vi "Tree -- Cron Library.vi"() -> ()   [LabVIEW 2013]
uses:
  JobReport/JobReport.lvclass
  JobReport/JobReport.lvclass/JobReport.ctl
  Job/Job Report -- cluster.ctl
  Job/Job.lvclass
  Job/Job.lvclass/Job.ctl
  Cron.Quartz/Cron.Quartz.lvclass
  Cron.Unix/Cron.Unix.lvclass
  Cron.Jenkins/Cron.Jenkins.lvclass
  Cron/Cron.lvclass/Cron.ctl
  Job/Read Abort Notifier.vi
  <vilib>/Utility/error.llb/Error Cluster From Error Code.vi
  Cron/Cron.lvclass
  openCron.lvlib
  Job.StaticVIRef/Job.StaticVIRef.lvclass
panel:
  out "Next Occurence 3":timestamp
  out "syntax valid? (Jenkins)":bool
  out "Next Occurence 2":timestamp
  out "syntax valid? (Unix)":bool
  out "syntax valid? (Quartz)":bool
  out "Next Occurence":timestamp
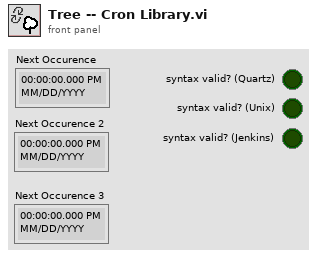
[diagram p1: front panel]
types:
  T1 = typedef "openCronJob.lvlib/JobReport.lvclass/Job Report -- cluster.ctl" = cluster{"Name":string, "GUID":string, "Start Time":timestamp, "Duration (s)":dbl, "exception code":i32, "stdin":string, "stdout":string}
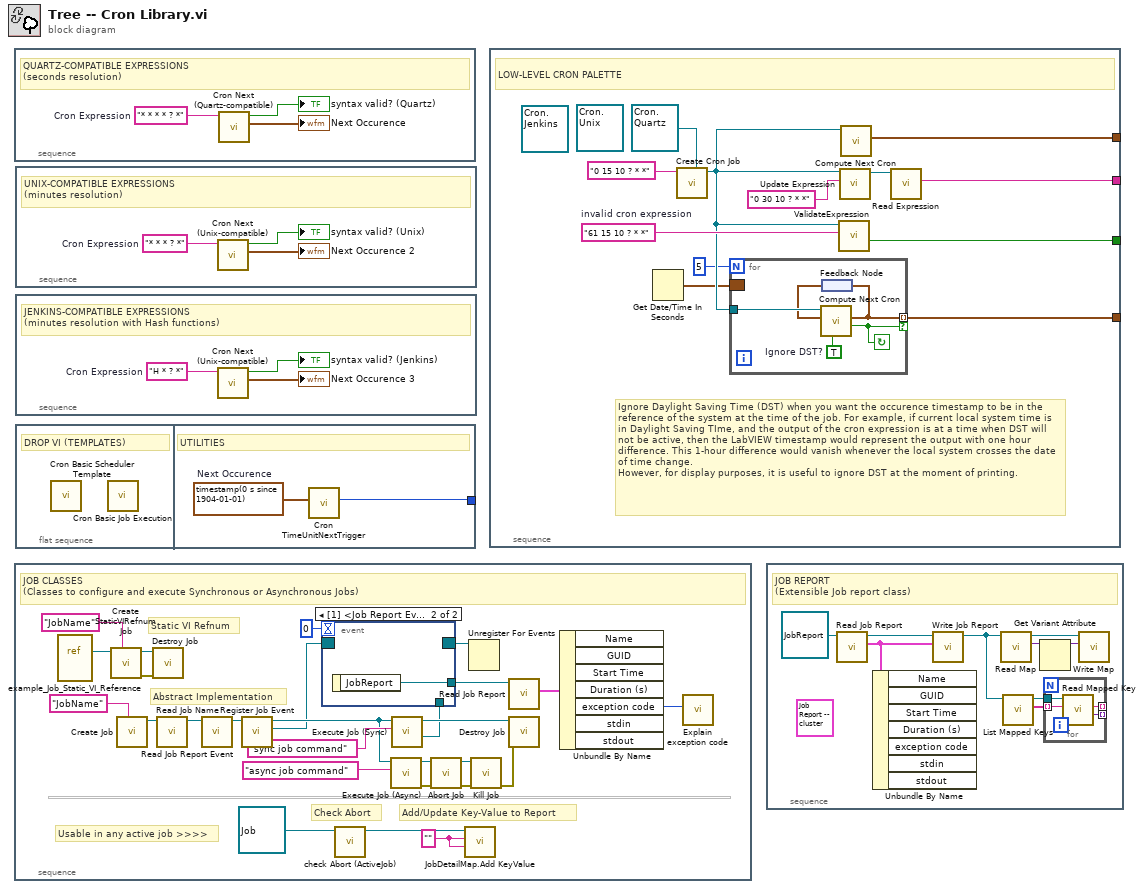
[diagram p0: block diagram]
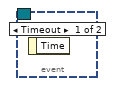
[diagram p2: hidden frame]
diagram:
  n1 = stacked-sequence {
    frame #0 {
      w3 = "* * * * ? *"  # Cron Expression
      # "QUARTZ-COMPATIBLE EXPRESSIONS\n(seconds resolution)"
      n2 = call "Cron Next (Quartz-compatible).vi"("Cron Expression"=w3) -> ("Next Occurence"=→"Next Occurence":timestamp, "syntax valid?"=→"syntax valid? (Quartz)":bool)  [unwired: 8 in, 1 out]
    }
  }
  n3 = stacked-sequence {
    frame #0 {
      w4 = "" ("Key")
      # "Add/Update Key-Value to Report"
      # "Check Abort"
      # "Usable in any active job >>>>"
      # "Abstract Implementation"
      # "Static VI Refnum"
      # "JOB CLASSES\n(Classes to configure and execute Synchronous or Asynchronous Jobs)"
      n4 = vi-ref "example_Job_Static_VI_Reference.vi"() -> (w14:refnum<vi>)
      n5 = call "Create StaticVIRefnum Job.vi"("Job Name"="JobName", "Static VI Refnum"=w14) -> ("error out"=w15:errorcluster, "Job.StaticVIRef out"=w16:refnum<class "Job.StaticVIRef.lvclass">)  [unwired: 8 in]
      n6 = call "Create Job.vi"("Job Name"="JobName") -> ("Job"=w29:refnum<class "Job.lvclass">)  [unwired: 9 in, 1 out]
      n7 = call "Destroy Job.vi"("error in (no error)"=w15, "Job in"=w16) -> ()  [unwired: 8 in, 2 out]
      n8 = call "Read Job Name.vi"("Job in"=w29) -> ("Job out"=w25:refnum<class "Job.lvclass">)  [unwired: 8 in, 2 out]
      n9 = call "Read Job Report Event.vi"("Job in"=w25) -> ("Job out"=w24:refnum<class "Job.lvclass">)  [unwired: 8 in, 2 out]
      n10 = call "Register Job Event.vi"("Job in"=w24) -> ("Job Event Registration"=w21:refnum<event-registration>, "Job out"=w26:refnum<class "Job.lvclass">)  [unwired: 9 in]
      n11 = call "check Abort (ActiveJob).vi"("Job in"=refnum<class "Job.lvclass"> refnum) -> ("Job out"=w5:refnum<class "Job.lvclass">)  [unwired: 7 in, 3 out]
      n12 = call "Execute Job (Async).vi"("stdin"="async job command" ("Job Name"), "Job in"=w26) -> ("error out"=w9:errorcluster, "Job out"=w23:refnum<class "Job.lvclass">)  [unwired: 7 in, 1 out]
      n13 = call "Execute Job (Sync).vi"("stdin"="sync job command" ("Job Name"), "Job in"=w26) -> ("JobReport"=w12:refnum<class "JobReport.lvclass">, "Job out"=w18:refnum<class "Job.lvclass">)  [unwired: 6 in, 2 out]
      n14 = event shown="[1] <Job Report Event>: User Event" {
        selector: w21 -> [_ _]
        dyn-events: [_ _] -> w20
        timeout: 0 -> [_ _]
        tunnel: [_ w31] -> w7
        tunnel: w12 -> [_ _]
        event Timeout {
          n15 = event-data() -> ()  [unwired: 1 in, 1 out]
        }
        event User Event {
          n16 = event-data() -> ("JobReport"=w31:refnum<class "JobReport.lvclass">)  [unwired: 1 in]
        }
      }
      n17 = call "Abort Job.vi"("error in (no error)"=w9, "Job in"=w23) -> ("error out"=w10:errorcluster, "Job out"=w22:refnum<class "Job.lvclass">)  [unwired: 5 in, 3 out]
      n18 = call "JobDetailMap.Add KeyValue.vi"("Value"=w4, "Key"=w4, "Job in"=w5) -> ()  [unwired: 7 in, 2 out]
      n19 = Unregister For Events(event registration refnum=w20) -> ()  [unwired: 1 in, 1 out]
      n20 = call "Kill Job.vi"("error in (no error)"=w10, "Job in"=w22) -> ("error out"=w11:errorcluster)  [unwired: 8 in, 1 out]
      n21 = call "Read Job Report.vi"("JobReport in"=w7) -> ("Job Report"=w8:T1)  [unwired: 8 in, 2 out]
      n22 = call "Destroy Job.vi"("error in (no error)"=w11, "Job in"=w18) -> ()  [unwired: 8 in, 2 out]
      n23 = Unbundle By Name(w8) -> ("exception code"=w17:i32)  [unwired: 6 out]
      n24 = call "Explain exception code.vi"("exception"=w17) -> ()  [unwired: 8 in, 3 out]
    }
  }
  n25 = stacked-sequence {
    frame #0 {
      w34 = "* * * ? *"  # Cron Expression
      # "UNIX-COMPATIBLE EXPRESSIONS\n(minutes resolution)"
      n26 = call "Cron Next (Unix-compatible).vi"("Cron Expression"=w34) -> ("Next Occurence"=→"Next Occurence 2":timestamp, "syntax valid?"=→"syntax valid? (Unix)":bool)  [unwired: 8 in, 1 out]
    }
  }
  n27 = stacked-sequence {
    frame #0 {
      w37 = "H * ? *"  # Cron Expression
      # "JENKINS-COMPATIBLE EXPRESSIONS\n(minutes resolution with Hash functions)"
      n28 = call "Cron Next (Unix-compatible).vi"("Cron Expression"=w37) -> ("Next Occurence"=→"Next Occurence 3":timestamp, "syntax valid?"=→"syntax valid? (Jenkins)":bool)  [unwired: 8 in, 1 out]
    }
  }
  n29 = flat-sequence {
    tunnel: [w38] -> _
    frame #0 {
      # "DROP VI (TEMPLATES)"
      n30 = call "Cron Basic Scheduler Template.vi"() -> ()  [unwired: 12 in]
      n31 = call "Cron Basic Job Execution.vi"() -> ()  [unwired: 12 in]
    }
    frame #1 {
      w39 = timestamp(0 s since 1904-01-01)  # Next Occurence
      # "UTILITIES"
      n32 = call "Cron TimeUnitNextTrigger.vi"("Next Occurence"=w39) -> ("next event (ms)"=w38:i32)  [unwired: 10 in]
    }
  }
  n33 = stacked-sequence {
    tunnel: [w43] -> _
    tunnel: [w42] -> _
    tunnel: [w41] -> _
    tunnel: [w40] -> _
    frame #0 {
      (unwired) refnum<class "Cron.Jenkins.lvclass"> refnum ("Cron.Jenkins")
      w49 = "61 15 10 ? * *"  # invalid cron expression
      (unwired) refnum<class "Cron.Unix.lvclass"> refnum ("openCron.lvlib:Cron.Unix.lvclass")
      # "Ignore Daylight Saving Time (DST) when you want the occurence timestamp to be in the reference of the system at the time of the job. For example, if current local system time is in Daylight Saving TIme, and the output of the cron expression is at a time when DST will not be active, then the LabVIEW timestamp would represent the output with one hour difference. This 1-hour difference would vanish whenever the local system crosses the date of time change.\nHowever, for display purposes, it is useful to ignore DST at the moment of printing."
      # "LOW-LEVEL CRON PALETTE"
      n34 = Get Date/Time In Seconds() -> (seconds since 1Jan1904=w45:timestamp)
      n35 = call "Create Cron Job.vi"("Cron in"=refnum<class "Cron.Quartz.lvclass"> refnum ("openCron.lvlib:Cron.Quartz.lvclass"), "Cron Expression"="0 15 10 ? * *") -> ("Cron out"=w46:refnum<class "Cron.Quartz.lvclass">)  [unwired: 7 in, 2 out]
      n36 = for {
        N: 5 -> [_]
        tunnel: [w54] -> w41 mode=indexing if=w56
        tunnel: w46 -> [w55]
        border: w45 -> [_]
        stop <- w56 continue-if-true
        w52 = TRUE  # Ignore DST?
        n37 = feedback #1() -> (w53:timestamp)
        n38 = call "Compute Next Cron.vi"("Ignore DST?"=w52, "Time Stamp (Now)"=w53, "Cron in"=w55) -> ("Occurence found"=w56:bool, "Next Occurence"=w54:timestamp)  [unwired: 5 in, 2 out]
        n39 = feedback-in #1(w54) -> ()
      }
      n40 = call "ValidateExpression.vi"("Expression"=w49, "Cron in"=w46) -> ("valid?"=w40:bool)  [unwired: 6 in, 3 out]
      n41 = call "Update Expression.vi"("Expression"="0 30 10 ? * *", "Cron in"=w46) -> ("Cron out"=w47:refnum<class "Cron.Quartz.lvclass">)  [unwired: 7 in, 2 out]
      n42 = call "Compute Next Cron.vi"("Cron in"=w46) -> ("Next Occurence"=w42:timestamp)  [unwired: 7 in, 3 out]
      n43 = call "Read Expression.vi"("Cron in"=w47) -> ("Expression"=w43:string)  [unwired: 8 in, 2 out]
    }
  }
  n44 = stacked-sequence {
    frame #0 {
      (unwired) T1 {"Name"="", "GUID"="", "Start Time"=timestamp(0 s since 1904-01-01), "Duration (s)"=0.0, "exception code"=0, "stdin"="", "stdout"=""} ("Job Report")
      # "JOB REPORT\n(Extensible Job report class)"
      n45 = call "Read Job Report.vi"("JobReport in"=refnum<class "JobReport.lvclass"> refnum ("openCronJob.lvlib:JobReport.lvclass")) -> ("Job Report"=w63:T1, "JobReport out"=w64:refnum<class "JobReport.lvclass">)  [unwired: 8 in, 1 out]
      n46 = Unbundle By Name(w63) -> ()  [unwired: 7 out]
      n47 = call "Write Job Report.vi"("Job Report"=w63, "JobReport in"=w64) -> ("JobReport out"=w59:refnum<class "JobReport.lvclass">)  [unwired: 8 in, 1 out]
      n48 = call "Read Map.vi"("JobReport in"=w59) -> ("Map"=w61:variant, "JobReport out"=w62:refnum<class "JobReport.lvclass">)  [unwired: 8 in, 1 out]
      n49 = call "List Mapped Keys.vi"("JobReport in"=w59) -> ("Mapped Keys"=w57:string[], "JobReport out"=w58:refnum<class "JobReport.lvclass">)  [unwired: 8 in, 1 out]
      n50 = Get Variant Attribute(Variant=w61) -> (duplicate Variant=w60:variant)  [unwired: 3 in, 3 out]
      n51 = for {
        tunnel: w58 -> [w69]
        tunnel: w57 -> [w68] mode=indexing
        tunnel: [w67] -> _ mode=indexing
        tunnel: [w66] -> _ mode=indexing
        n52 = call "Read Mapped Key.vi"("Key"=w68, "JobReport in"=w69) -> ("Value"=w66:variant, "Key dup"=w67:string)  [unwired: 5 in, 3 out]
      }
      n53 = call "Write Map.vi"("Map"=w60, "JobReport in"=w62) -> ()  [unwired: 8 in, 2 out]
    }
  }
